vi "ConvertToDecimal.vi"(1 "read buffer":string) -> (0 "unsigned byte array":u8[](array[numeric]))   [LabVIEW 2017, in "Spectral Products CM110.lvlib"]
uses:
  Spectral Products CM110.lvlib
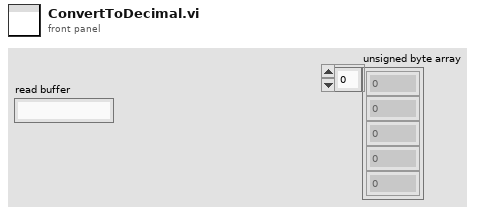
[diagram p1: front panel]
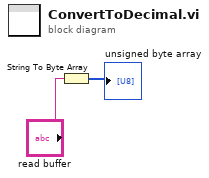
[diagram p0: block diagram]
diagram:
  n1 = String To Byte Array(string="read buffer") -> (unsigned byte array=→"unsigned byte array":u8[])
